vi "Write Mission Controller State Msg.vi"(8 "error in (no error)":errorcluster, 10 "Mission Controller State":T1 {"Mission"."GPS Longitude" format="%.6g"; "Mission"."GPS Latitude" format="%.6g"}, 11 "Mission Controller State Message in":refnum<class "Mission Controller State Message.lvclass">) -> (0 "error out":errorcluster, 3 "Mission Controller State Message out":refnum<class "Mission Controller State Message.lvclass">)   [LabVIEW 2015, in "RDS Child Messages.lvlib" / "Mission Controller State Message.lvclass"]
uses:
  Mission Controller State Message.lvclass
  Mission Controller State Control.ctl
  RDS Mission Controller Actor/Mission Controller Navigation State.ctl
  RDS Mission Controller Actor/MissionOp.ctl
  Mission Controller State Message.lvclass/Mission Controller State Message.ctl
  RDS Mission Controller Actor/RDS Mission Controller Actor.lvlib
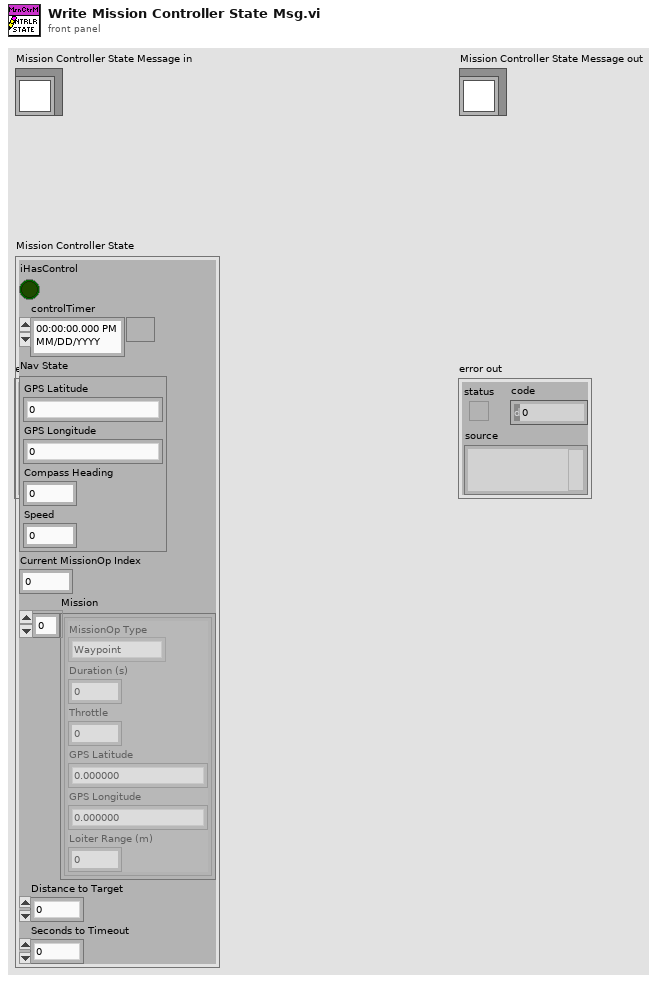
[diagram p1: front panel]
types:
  T1 = typedef "RDS Child Messages.lvlib/Mission Controller State Message.lvclass/Mission Controller State Control.ctl" = cluster{"iHasControl":bool, "controlTimer":timestamp, "Nav State":T2, "Current MissionOp Index":i32, "Mission":T3[], "Distance to Target":dbl, "Seconds to Timeout":dbl}
  T2 = typedef "RDS Mission Controller Actor.lvlib/Mission Controller Navigation State.ctl" = cluster{"GPS Latitude":ext, "GPS Longitude":ext, "Compass Heading":dbl, "Speed":dbl}
  T3 = typedef "RDS Mission Controller Actor.lvlib/MissionOp.ctl" = cluster{"MissionOp Type":enum16{"Waypoint", "Loiter", "Wait", "Deploy AIP", "Stow AIP"}, "Duration (s)":u16, "Throttle":i16, "GPS Latitude":dbl, "GPS Longitude":dbl, "Loiter Range (m)":u16}
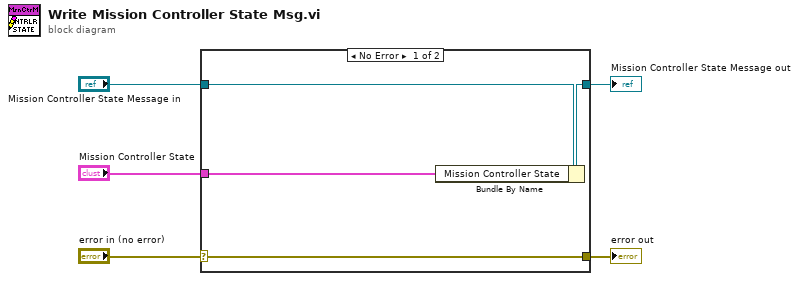
[diagram p0: block diagram]
diagram:
  n1 = case shown="No Error" "error in (no error)" {
    selector: "error in (no error)" -> [w9 w10]
    tunnel: [w9 w10] -> w4
    tunnel: [w7 w11] -> w2
    tunnel: "Mission Controller State Message in" -> [w8 w11]
    tunnel: "Mission Controller State" -> [w6 _]
    frame No Error {
      n2 = Bundle By Name(cluster=w8, "Mission Controller State"=w6) -> (w7:refnum<class "Mission Controller State Message.lvclass">)
    }
    frame Error {
    }
  }
  "error out" <- w4
  "Mission Controller State Message out" <- w2
